vi "Command Type.vi"(11 "Numeric Command Config in":refnum<class "Numeric Command Config.lvclass">) -> (2 "Command Type":string)   [LabVIEW 2020, in "VolatusSeqConfig.lvlib" / "Numeric Command Config.lvclass"]
uses:
  Numeric Command Config.lvclass
  Numeric Command Config.lvclass/Numeric Command Config.ctl
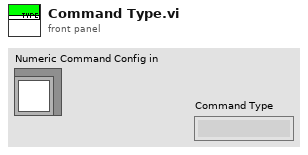
[diagram p1: front panel]
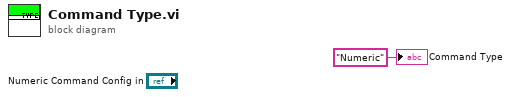
[diagram p0: block diagram]
diagram:
  "Command Type" <- "Numeric" ("Command Type")
